vi "Area of Triangle.vi"(1 "C边(cm)":dbl, 2 "B边(cm)":dbl, 3 "A边(cm)":dbl) -> (0 "三角形面积(cm^2)":dbl)   [LabVIEW 2012]
doc: "本VI使用海伦公式计算三角形面积：\n\n面积＝(s * (s-a) * (s-b) * (s-c))的平方根\n\ns＝(a+b+c)/2；a、b、c为三角形的边。"
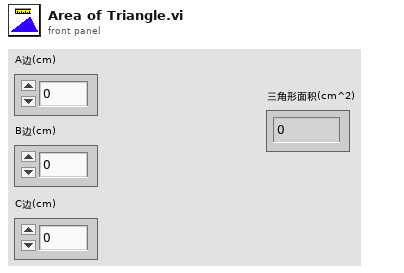
[diagram p1: front panel]
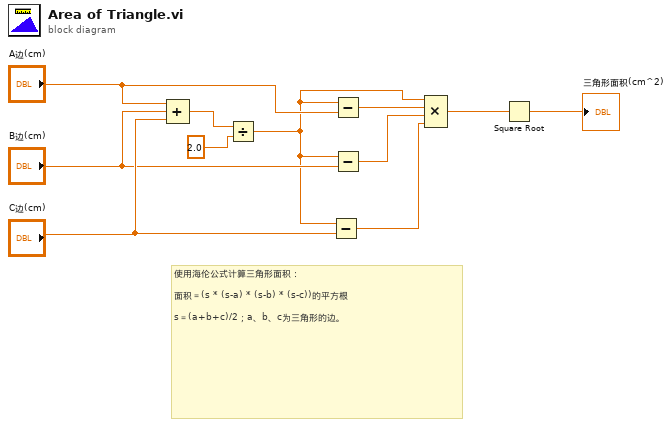
[diagram p0: block diagram]
diagram:
  # "使用海伦公式计算三角形面积：\n\n面积＝(s * (s-a) * (s-b) * (s-c))的平方根\n\ns＝(a+b+c)/2；a、b、c为三角形的边。"
  n1 = Compound Arithmetic op=ADD ("复合运算")("A边(cm)", "B边(cm)", "C边(cm)") -> (w4:dbl)
  n2 = Divide ("除")(x=w4, y=2.0) -> (x/y=w1:dbl)
  n3 = Subtract ("减")(x=w1, y="C边(cm)") -> (x-y=w7:dbl)
  n4 = Subtract ("减")(x=w1, y="A边(cm)") -> (x-y=w9:dbl)
  n5 = Subtract ("减")(x=w1, y="B边(cm)") -> (x-y=w8:dbl)
  n6 = Compound Arithmetic op=MULTIPLY ("复合运算")(w1, w9, w8, w7) -> (w6:dbl)
  n7 = Square Root ("平方根")(x=w6) -> (sqrt(x)=→"三角形面积(cm^2)":dbl)
